vi "niDTS BT INSTR RX Configure BT Basic Parameters.vi"(8 "error in (no error)":errorcluster, 11 "niDTS BT INSTR RX in":refnum<class "niDTS BT INSTR RX.lvclass">) -> (0 "error out":errorcluster, 3 "niDTS BT INSTR RX out":refnum<class "niDTS BT INSTR RX.lvclass">)   [LabVIEW 2015, in "niDTS BT.lvlib" / "niDTS BT INSTR RX.lvclass"]
uses:
  niDTS BT INSTR RX.lvclass
  niDTS BT INSTR RX.lvclass/niDTS BT INSTR RX.ctl
  RiviInstDriver/niRfsgBT/Objects/niRfsgBt.lvclass
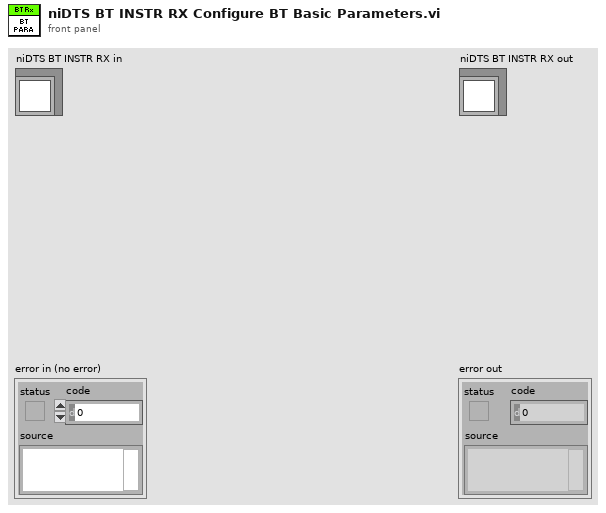
[diagram p1: front panel]
types:
  T1 = cluster{"PacketType":enum16{"NULL", "POLL", "FHS", "DH1", "DH3", "DH5", "DM1", "DM3", "DM5", "HV1", "HV2", "HV3", "EV3", "EV4", "EV5", "DV", "AUX1", "LETP"}, "PacketPayloadDataRate":i32}
  T2 = enum16{"NULL", "POLL", "FHS", "DH1", "DH3", "DH5", "DM1", "DM3", "DM5", "HV1", "HV2", "HV3", "EV3", "EV4", "EV5", "DV", "AUX1", "LETP"}
  T3 = typedef "niRfsgBT.lvclass/niRfsgBT INC Handle.ctl" = refnum<data-value>
  T4 = typedef "niDTS BT.lvlib/niDTS BT INC Packet Type.ctl" = enum16{"NULL", "POLL", "FHS", "DM1", "DH1", "HV1", "HV2", "HV3", "EV3", "DV", "AUX1", "DM3", "DH3", "EV4", "EV5", "DM5", "DH5", "LE-TP"}
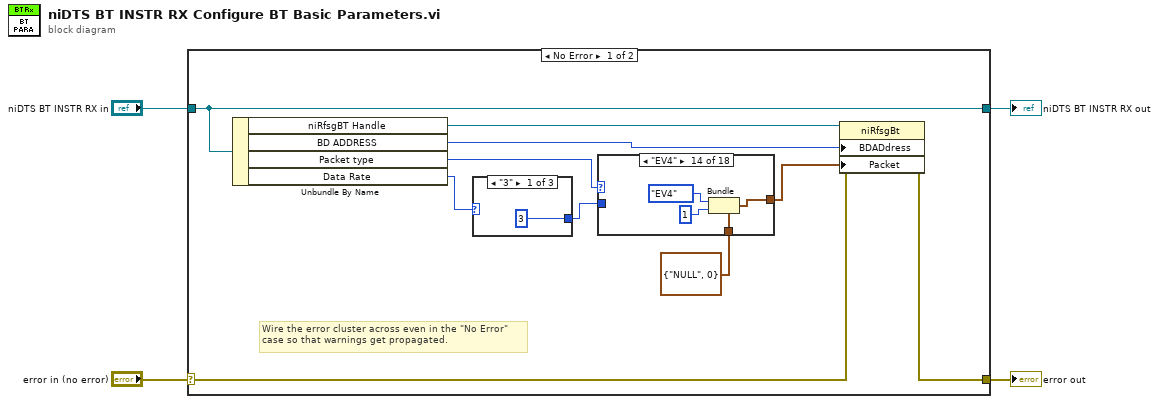
[diagram p0: block diagram]
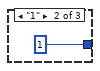
[diagram p2: hidden frame]
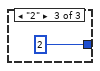
[diagram p3: hidden frame]
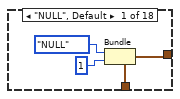
[diagram p4: hidden frame]
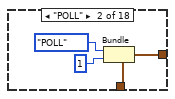
[diagram p5: hidden frame]
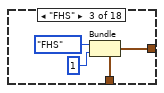
[diagram p6: hidden frame]
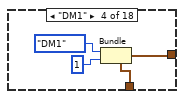
[diagram p7: hidden frame]
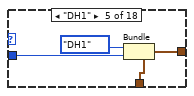
[diagram p8: hidden frame]
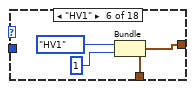
[diagram p9: hidden frame]
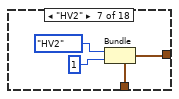
[diagram p10: hidden frame]
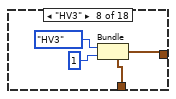
[diagram p11: hidden frame]
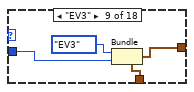
[diagram p12: hidden frame]
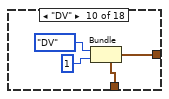
[diagram p13: hidden frame]
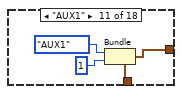
[diagram p14: hidden frame]
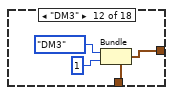
[diagram p15: hidden frame]
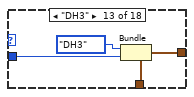
[diagram p16: hidden frame]
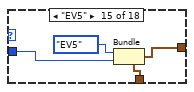
[diagram p17: hidden frame]
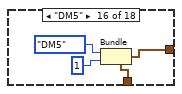
[diagram p18: hidden frame]
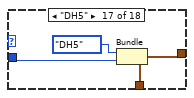
[diagram p19: hidden frame]
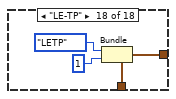
[diagram p20: hidden frame]
diagram:
  n1 = case shown="No Error" "error in (no error)" {
    selector: "error in (no error)" -> [w11 w91]
    tunnel: [w10 w91] -> w3
    tunnel: [w14 w90] -> w1
    tunnel: "niDTS BT INSTR RX in" -> [w14 w90]
    frame No Error {
      # "Wire the error cluster across even in the \"No Error\"\ncase so that warnings get propagated."
      n2 = Unbundle By Name(w14) -> ("niRfsgBT Handle"=w13:T3, "BD ADDRESS"=w12:i64, "Packet type"=w9:T4, "Data Rate"=w6:enum16{"1", "2", "3"})
      n3 = case shown="\"3\"" w6 {
        tunnel: [3 ("Data Rate") 1 ("Data Rate") 2 ("Data Rate")] -> w5
        frame "3" {
        }
        frame "1" {
        }
        frame "2" {
        }
      }
      n4 = case shown="\"EV4\"" w9 {
        tunnel: w5 -> [_ _ _ _ w34 _ _ _ w50 _ _ _ w68 _ w75 _ w84 _]
        tunnel: T1 {"PacketType"=enum."NULL", "PacketPayloadDataRate"=0} ("SOURce:RFSG:BLUetooth:Packet") -> [w19 w23 w27 w31 w35 w39 w43 w47 w52 w55 w59 w63 w67 w71 w76 w79 w83 w89]
        tunnel: [w18 w22 w26 w30 w36 w38 w42 w46 w51 w54 w58 w62 w66 w70 w74 w78 w82 w88] -> w7
        frame "NULL", Default {
          n5 = Bundle(cluster=w19, "PacketType"=T2."NULL", "PacketPayloadDataRate"=1) -> (w18:T1)
        }
        frame "POLL" {
          n6 = Bundle(cluster=w23, "PacketType"=T2."POLL", "PacketPayloadDataRate"=1) -> (w22:T1)
        }
        frame "FHS" {
          n7 = Bundle(cluster=w27, "PacketType"=T2."FHS", "PacketPayloadDataRate"=1) -> (w26:T1)
        }
        frame "DM1" {
          n8 = Bundle(cluster=w31, "PacketType"=T2."DM1", "PacketPayloadDataRate"=1) -> (w30:T1)
        }
        frame "DH1" {
          n9 = Bundle(cluster=w35, "PacketType"=T2."DH1", "PacketPayloadDataRate"=w34) -> (w36:T1)
        }
        frame "HV1" {
          n10 = Bundle(cluster=w39, "PacketType"=T2."HV1", "PacketPayloadDataRate"=1) -> (w38:T1)
        }
        frame "HV2" {
          n11 = Bundle(cluster=w43, "PacketType"=T2."HV2", "PacketPayloadDataRate"=1) -> (w42:T1)
        }
        frame "HV3" {
          n12 = Bundle(cluster=w47, "PacketType"=T2."HV3", "PacketPayloadDataRate"=1) -> (w46:T1)
        }
        frame "EV3" {
          n13 = Bundle(cluster=w52, "PacketType"=T2."EV3", "PacketPayloadDataRate"=w50) -> (w51:T1)
        }
        frame "DV" {
          n14 = Bundle(cluster=w55, "PacketType"=T2."DV", "PacketPayloadDataRate"=1) -> (w54:T1)
        }
        frame "AUX1" {
          n15 = Bundle(cluster=w59, "PacketType"=T2."AUX1", "PacketPayloadDataRate"=1) -> (w58:T1)
        }
        frame "DM3" {
          n16 = Bundle(cluster=w63, "PacketType"=T2."DM3", "PacketPayloadDataRate"=1) -> (w62:T1)
        }
        frame "DH3" {
          n17 = Bundle(cluster=w67, "PacketType"=T2."DH3", "PacketPayloadDataRate"=w68) -> (w66:T1)
        }
        frame "EV4" {
          n18 = Bundle(cluster=w71, "PacketType"=T2."EV4", "PacketPayloadDataRate"=1) -> (w70:T1)
        }
        frame "EV5" {
          n19 = Bundle(cluster=w76, "PacketType"=T2."EV5", "PacketPayloadDataRate"=w75) -> (w74:T1)
        }
        frame "DM5" {
          n20 = Bundle(cluster=w79, "PacketType"=T2."DM5", "PacketPayloadDataRate"=1) -> (w78:T1)
        }
        frame "DH5" {
          n21 = Bundle(cluster=w83, "PacketType"=T2."DH5", "PacketPayloadDataRate"=w84) -> (w82:T1)
        }
        frame "LE-TP" {
          n22 = Bundle(cluster=w89, "PacketType"=T2."LETP", "PacketPayloadDataRate"=1) -> (w88:T1)
        }
      }
      n23 = property class="niRfsgBt"(reference=w13, error in=w11, "BDADdress"=w12, "Packet"=w7) -> (error out=w10:errorcluster)  [unwired: 1 out]
    }
    frame Error {
    }
  }
  "error out" <- w3
  "niDTS BT INSTR RX out" <- w1
